vi "Keithley 6514 Initiate-Abort.vi"(0 "Resource In":refnum<visa-resource-name>, 7 "Action (Init One Cycle:0)":u32(knob) scale=0.0..1.0, 11 "error in (no error)":T1) -> (4 "Resource Out (dupl)":refnum<visa-resource-name>, 15 "error out":T1)   [LabVIEW 2009, in "Keithley 6514 LV 2009.lvlib"]
doc: "This VI for the Keithley 6514 allows the operator to Initiate Triggering or Abort Triggering.\n\nInitiate/Abort:\n0 = Initiate One Cycle\n1 = Abort Triggering"
uses:
  Keithley 6514 LV 2009.lvlib
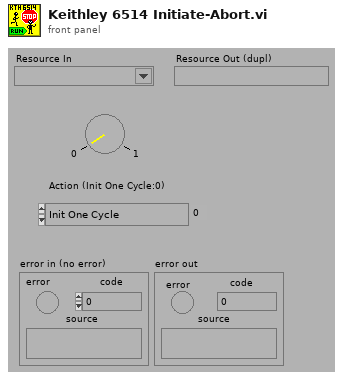
[diagram p1: front panel]
types:
  T1 = cluster{"error":bool, "code":i32, "source":string}
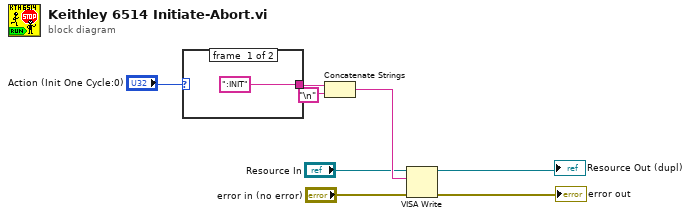
[diagram p0: block diagram]
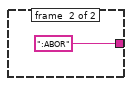
[diagram p2: hidden frame]
diagram:
  n1 = case shown="1" "Action (Init One Cycle:0)" {
    tunnel: [":INIT" ":ABOR"] -> w7
    frame #0 {
    }
    frame #1 {
    }
  }
  n2 = Concatenate Strings(w7, "\n") -> (w5:string)
  n3 = VISA Write(VISA resource name="Resource In", write buffer=w5, error in (no error)="error in (no error)") -> (VISA resource name out=→"Resource Out (dupl)":refnum<visa-resource-name>, error out=→"error out":errorcluster)  [unwired: 1 out]
